vi "Generator DC Sweep Manager.vi"(8 "error in (no error)":errorcluster, 10 "sweep state":T1=enum."sweep", 11 "Generator in":refnum<class "Generator.lvclass">) -> (0 "error out":errorcluster, 2 "Waveform []":waveform(dbl)[](array[waveform]), 3 "Generator out":refnum<class "Generator.lvclass">)   [LabVIEW 2019, in "Generator.lvclass"]
uses:
  Generator.lvclass
  Instrument.DAQ/Typedefs/Sweep.State--enum.ctl
  Instrument.DAQ/Instrument.DAQ.lvclass
panel:
  out "time":dbl
  out "sweeping":dbl
  out "start sweep time":timestamp
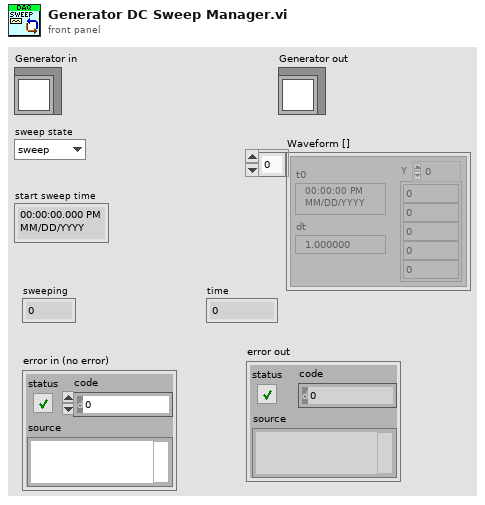
[diagram p1: front panel]
types:
  T1 = typedef "Instrument.Lockin.lvlib/Instrument.DAQ.lvclass/Sweep.State--enum.ctl" = enum16{"idle", "initialize", "wait", "sweep", "stop"}
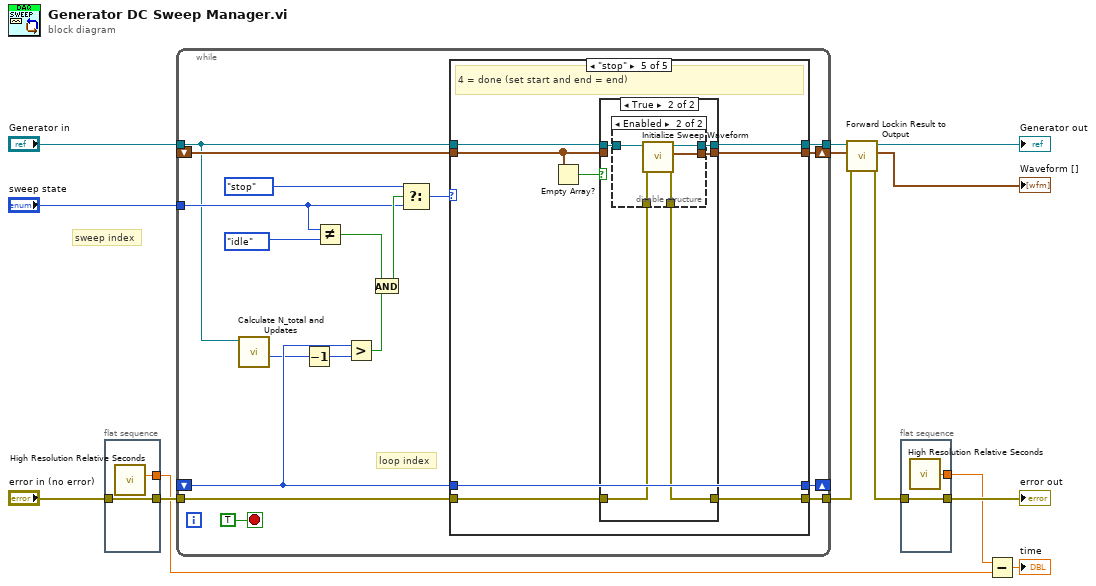
[diagram p0: block diagram]
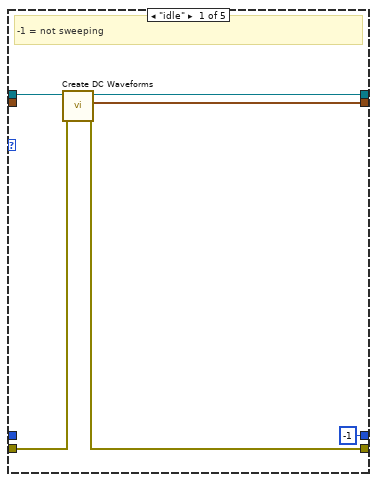
[diagram p2: hidden frame]
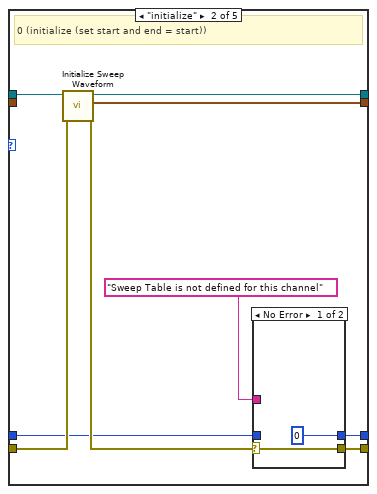
[diagram p3: hidden frame]
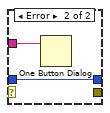
[diagram p4: hidden frame]
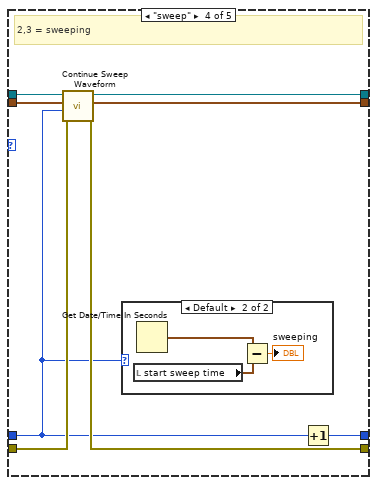
[diagram p6: hidden frame]
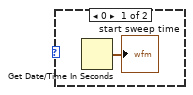
[diagram p7: hidden frame]
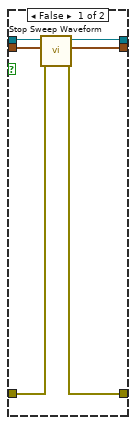
[diagram p8: hidden frame]
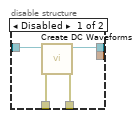
[diagram p9: hidden frame]
diagram:
  # "sweep index"
  n1 = flat-sequence {
    tunnel: "error in (no error)" -> [w16]
    tunnel: [w16] -> w11
    tunnel: [w15] -> w9
    frame #0 {
      n2 = call <vilib>:"High Resolution Relative Seconds.vi"() -> ("relative seconds"=w15:dbl)
    }
  }
  n3 = while {
    tunnel: "sweep state" -> [w24]
    shift-right: [w34] -> _
    shift-left: _ -> [w29]
    tunnel: [w32] -> w4
    tunnel: "Generator in" -> [w17]
    tunnel: w11 -> [w31]
    tunnel: [w30] -> w2
    shift-right: [w27] -> w3
    shift-left: _ -> [w18]
    stop <- TRUE stop-if-true
    # "loop index"
    n4 = call "Calculate N_total and Updates.vi"("Generator in"=w17) -> ("Updates"=w23:i32)  [unwired: 8 in, 2 out]
    n5 = Decrement(x=w23) -> (x-1=w22:i32)
    n6 = Not Equal?(x=w24, y=Sweep.State--enum."idle" ("sweep state")) -> (x != y?=w25:bool)
    n7 = Greater?(x=w29, y=w22) -> (0:w28:bool)
    n8 = And(x=w25, y=w28) -> (x .and. y?=w26:bool)
    n9 = Select(t=Sweep.State--enum."stop" ("sweep state"), s=w26, f=w24) -> (s? t:f=w21:T1)
    n10 = case shown="\"stop\"" w21 {
      tunnel: [-1 w49 w54 w65 w77] -> w34
      tunnel: w29 -> [_ w41 w54 w58 w77]
      tunnel: [w36 w44 w57 w62 w74] -> w32
      tunnel: w31 -> [w39 w46 w56 w60 w76]
      tunnel: [w38 w42 w56 w59 w73] -> w30
      tunnel: [w37 w45 w55 w61 w72] -> w27
      tunnel: w17 -> [w35 w47 w57 w64 w75]
      tunnel: w18 -> [_ _ w55 w63 w70]
      frame "idle" {
        # "-1 = not sweeping"
        n11 = call "Create DC Waveforms.vi"("error in (no error)"=w39, "Generator in"=w35) -> ("Error out"=w38:errorcluster, "Waveforms out"=w37:waveform(dbl)[], "Generator out"=w36:refnum<class "Generator.lvclass">)  [unwired: 7 in]
      }
      frame "initialize" {
        # "0 (initialize (set start and end = start))"
        n12 = call "Initialize Sweep Waveform.vi"("error in (no error)"=w46, "Generator in"=w47) -> ("error out"=w43:errorcluster, "Waveforms"=w45:waveform(dbl)[], "Generator out"=w44:refnum<class "Generator.lvclass">)  [unwired: 7 in]
        n13 = case shown="No Error" w43 {
          selector: w43 -> [w50 _]
          tunnel: [0 w53] -> w49
          tunnel: w41 -> [_ w53]
          tunnel: "Sweep Table is not defined for this channel" -> [_ w52]
          tunnel: [w50 _] -> w42
          frame No Error {
          }
          frame Error {
            n14 = One Button Dialog(message=w52) -> ()  [unwired: 1 in, 1 out]
          }
        }
      }
      frame "wait" {
        # "1 (waiting): do nothing"
      }
      frame "sweep" {
        # "2,3 = sweeping"
        n15 = call "Continue Sweep Waveform.vi"("error in (no error)"=w60, "Sweep Index"=w58, "Waveforms in"=w63, "Generator in"=w64) -> ("error out"=w59:errorcluster, "Waveforms out"=w61:waveform(dbl)[], "Generator in"=w62:refnum<class "Generator.lvclass">)  [unwired: 5 in]
        n16 = case shown="Default" w58 {
          frame 0 {
            n17 = Get Date/Time In Seconds() -> (seconds since 1Jan1904=→"start sweep time":timestamp)
          }
          frame Default {
            n18 = local read "start sweep time"() -> (w68:timestamp)
            n19 = Get Date/Time In Seconds() -> (seconds since 1Jan1904=w67:timestamp)
            n20 = Subtract(x=w67, y=w68) -> (x-y=→"sweeping":dbl)
          }
        }
        n21 = Increment(x=w58) -> (x+1=w65:i32)
      }
      frame "stop" {
        # "4 = done (set start and end = end)"
        n22 = Empty Array?(array=w70) -> (empty?=w71:bool)
        n23 = case shown="True" w71 {
          tunnel: w76 -> [w83 w86]
          tunnel: w75 -> [w82 w88]
          tunnel: [w81 w87] -> w74
          tunnel: [w80 w85] -> w73
          tunnel: [w79 w84] -> w72
          tunnel: w70 -> [w78 _]
          frame False {
            n24 = call "Stop Sweep Waveform.vi"("error in (no error)"=w83, "Waveforms in"=w78, "Generator in"=w82) -> ("error out"=w80:errorcluster, "Waveforms out"=w79:waveform(dbl)[], "Generator out"=w81:refnum<class "Generator.lvclass">)  [unwired: 6 in]
          }
          frame True {
            n25 = disable-structure shown="Enabled" {
              disable-tunnel: w88 -> [w92 w97]
              disable-tunnel: [w91 w96] -> w87
              disable-tunnel: w86 -> [w90 w93]
              disable-tunnel: [w89 w94] -> w85
              disable-tunnel: [_ w95] -> w84
              frame Disabled {
                n26 = call "Create DC Waveforms.vi"("error in (no error)"=w90, "Generator in"=w92) -> ("Error out"=w89:errorcluster, "Generator out"=w91:refnum<class "Generator.lvclass">)  [unwired: 7 in, 1 out]
              }
              frame Enabled {
                n27 = call "Initialize Sweep Waveform.vi"("error in (no error)"=w93, "Generator in"=w97) -> ("error out"=w94:errorcluster, "Waveforms"=w95:waveform(dbl)[], "Generator out"=w96:refnum<class "Generator.lvclass">)  [unwired: 7 in]
              }
            }
          }
        }
      }
    }
  }
  n28 = call "Forward Lockin Result to Output.vi"("error in (no error)"=w2, "Waveforms [] in"=w3, "Generator in"=w4) -> ("error out"=w6:errorcluster, "Waveforms [] out"=→"Waveform []":waveform(dbl)[], "Generator out"=→"Generator out":refnum<class "Generator.lvclass">)  [unwired: 6 in]
  n29 = flat-sequence {
    tunnel: w6 -> [w99]
    tunnel: [w99] -> w10
    tunnel: [w98] -> w7
    frame #0 {
      n30 = call <vilib>:"High Resolution Relative Seconds.vi"() -> ("relative seconds"=w98:dbl)
    }
  }
  n31 = Subtract(x=w7, y=w9) -> (x-y=→"time":dbl)
  "error out" <- w10
